vi "Anaysis Point Tool Histogram.vi"(0 "Pointer Listbox Detail":string[][](array[string]), 1 "Image":T1(plugin-control), 3 "Fixturing ROI":i32[](array[numeric]), 5 "error in":errorcluster) -> (14 "Pass/Fail":bool, 15 "Image":T1(plugin-control), 17 "Array":T2(array[cluster]), 19 "error out":errorcluster)   [LabVIEW 2020]
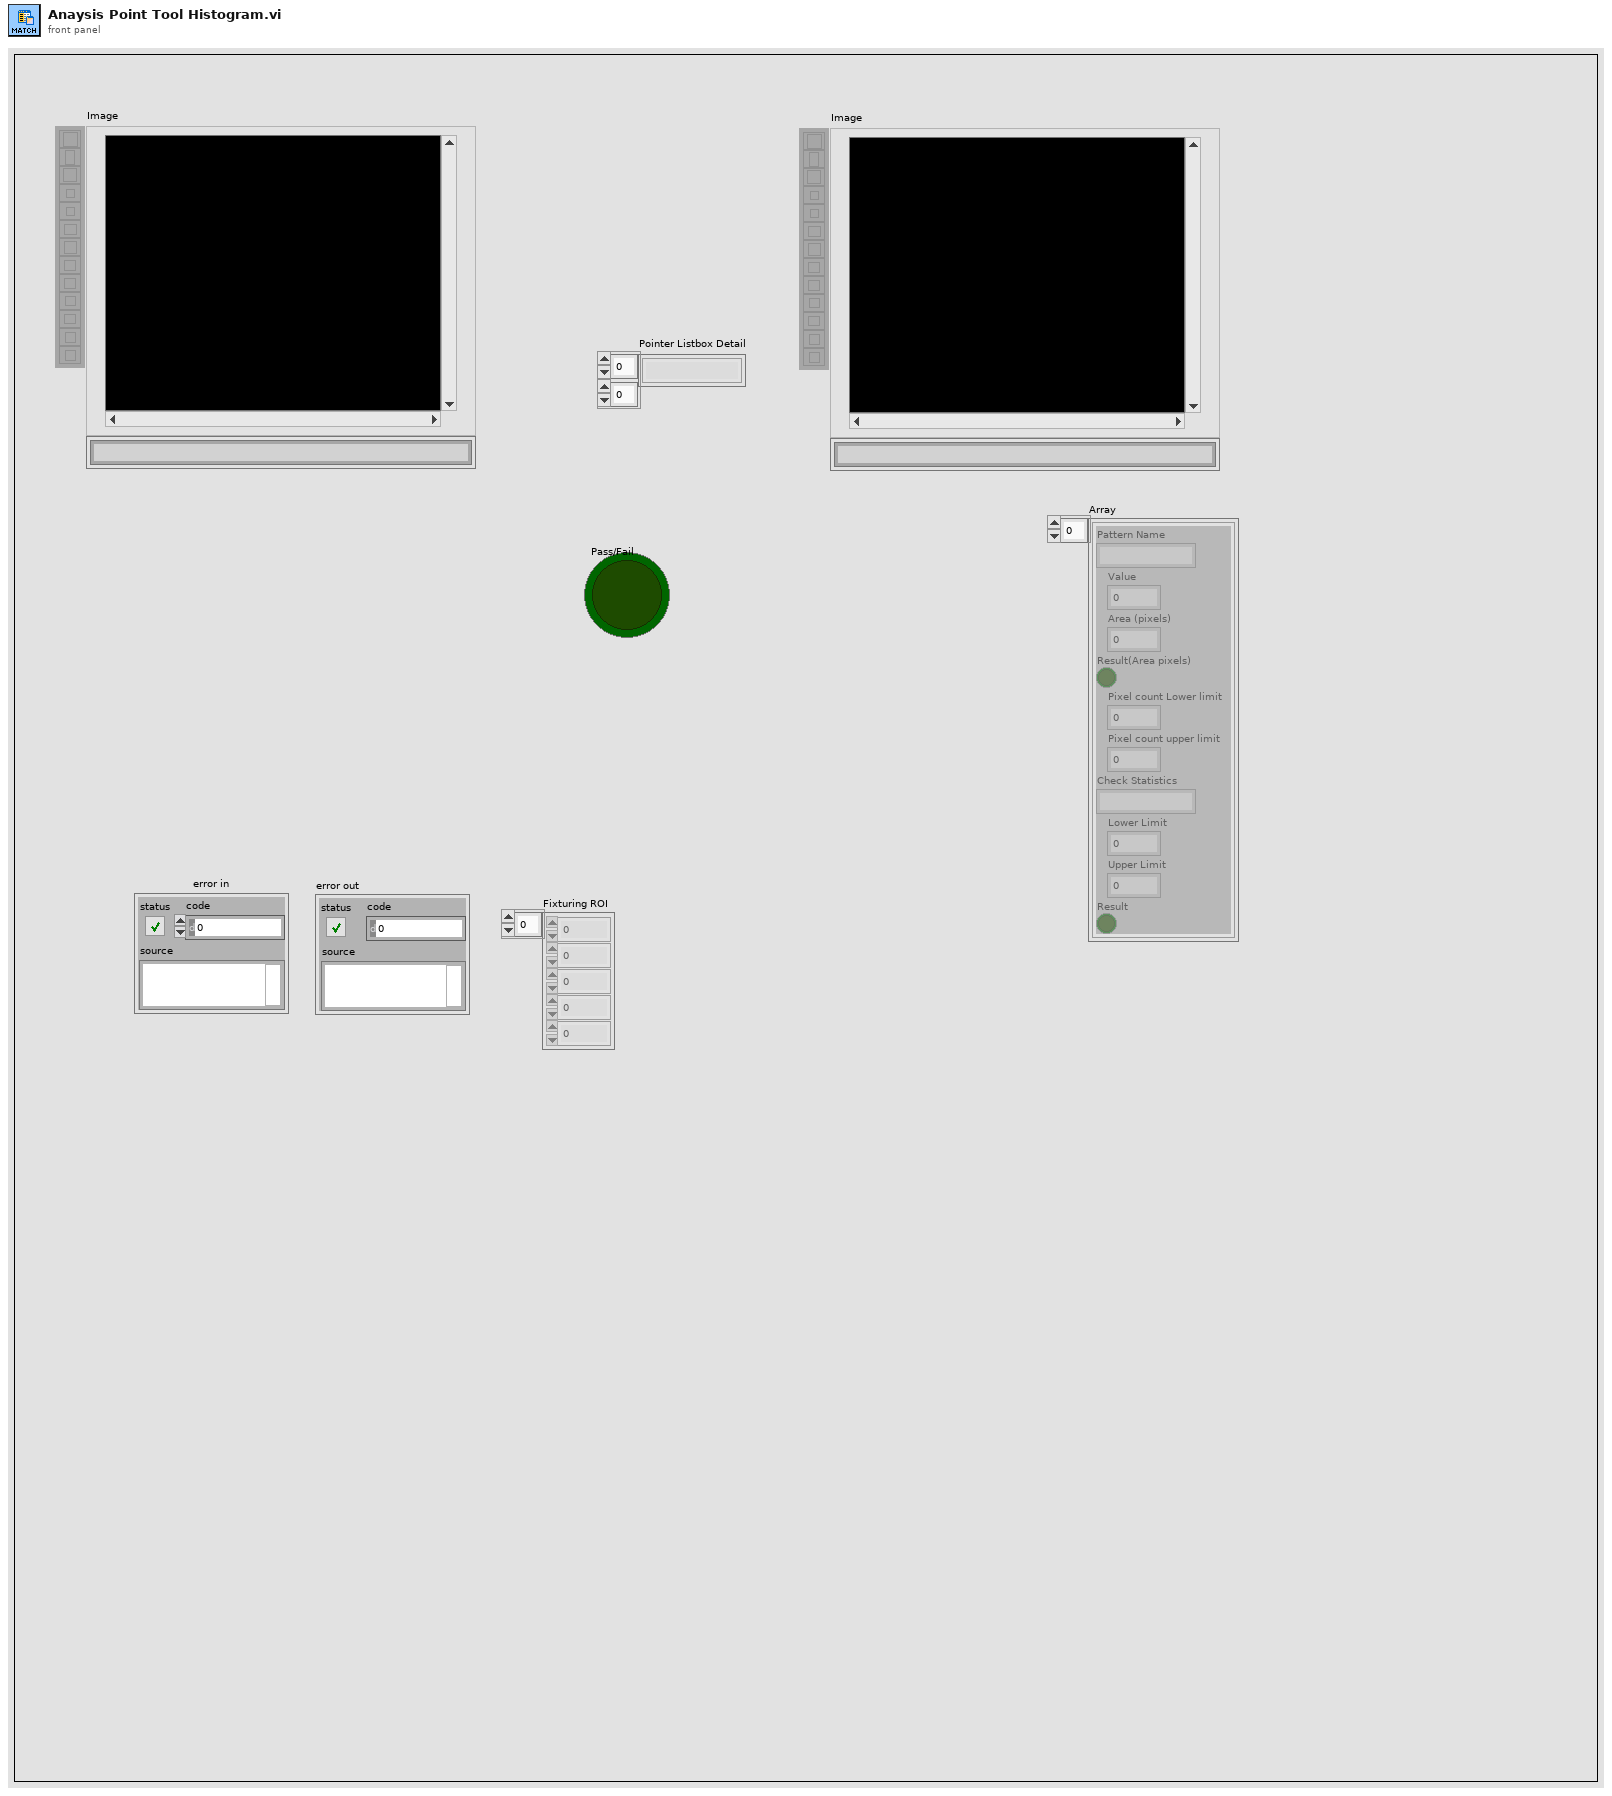
[diagram p1: front panel]
types:
  T1 = typedef "IMAQ Image.ctl" = refnum<image>
  T2 = cluster{"Pattern Name":string, "Value":ext, "Area (pixels)":i32, "Result(Area pixels)":bool, "Pixel count Lower limit":i32, "Pixel count upper limit":i32, "Check Statistics":string, "Lower Limit":i32, "Upper Limit":i32, "Result":bool}[]
  T3 = cluster{"Pixel count Lower limit":i32, "Pixel count upper limit":i32, "Check Statistics":string, "Lower Limit":i32, "Upper Limit":i32}
  T4 = cluster{"Global Rectangle":i32[], "Contours":cluster{"Contour Type":u32, "ROI Type":u32, "Points":i32[]}[]}
  T5 = cluster{"Global rect[0]":i32, "Global rect[1]":i32}
  T6 = cluster{i32[], cluster{"Contour Type":u32, "Contour Type":i32, i32[]}[]}
  T7 = cluster{"Minimal Value":sgl, "Maximal Value":sgl, "Mean Value":sgl, "Standard  Variation":sgl, "Area (pixels)":i32}
  T8 = typedef "ROI Descriptor" = cluster{"Global Rectangle":i32[], "Contours":cluster{"ID":enum32{"External", "Internal"}, "Type":u32, "Coordinates":i32[]}[]}
  T9 = cluster{"Rectangle out[0]":i32, "Rectangle out[1]":i32, "Rectangle out[2]":i32, "Rectangle out[3]":i32, "Rectangle out[4]":i32, "Rectangle out[5]":i32, "Rectangle out[6]":i32, "Rectangle out[7]":i32, "Rectangle out[8]":i32}
  T10 = cluster{"Rectangle out[0]":i32, "Rectangle out[1]":i32, "Rectangle out[2]":i32, "Rectangle out[3]":i32}
  T11 = cluster{"Pattern Name":string, "Value":ext, "Area (pixels)":i32, "Result(Area pixels)":bool, "Pixel count Lower limit":i32, "Pixel count upper limit":i32, "Check Statistics":string, "Lower Limit":i32, "Upper Limit":i32, "Result":bool}
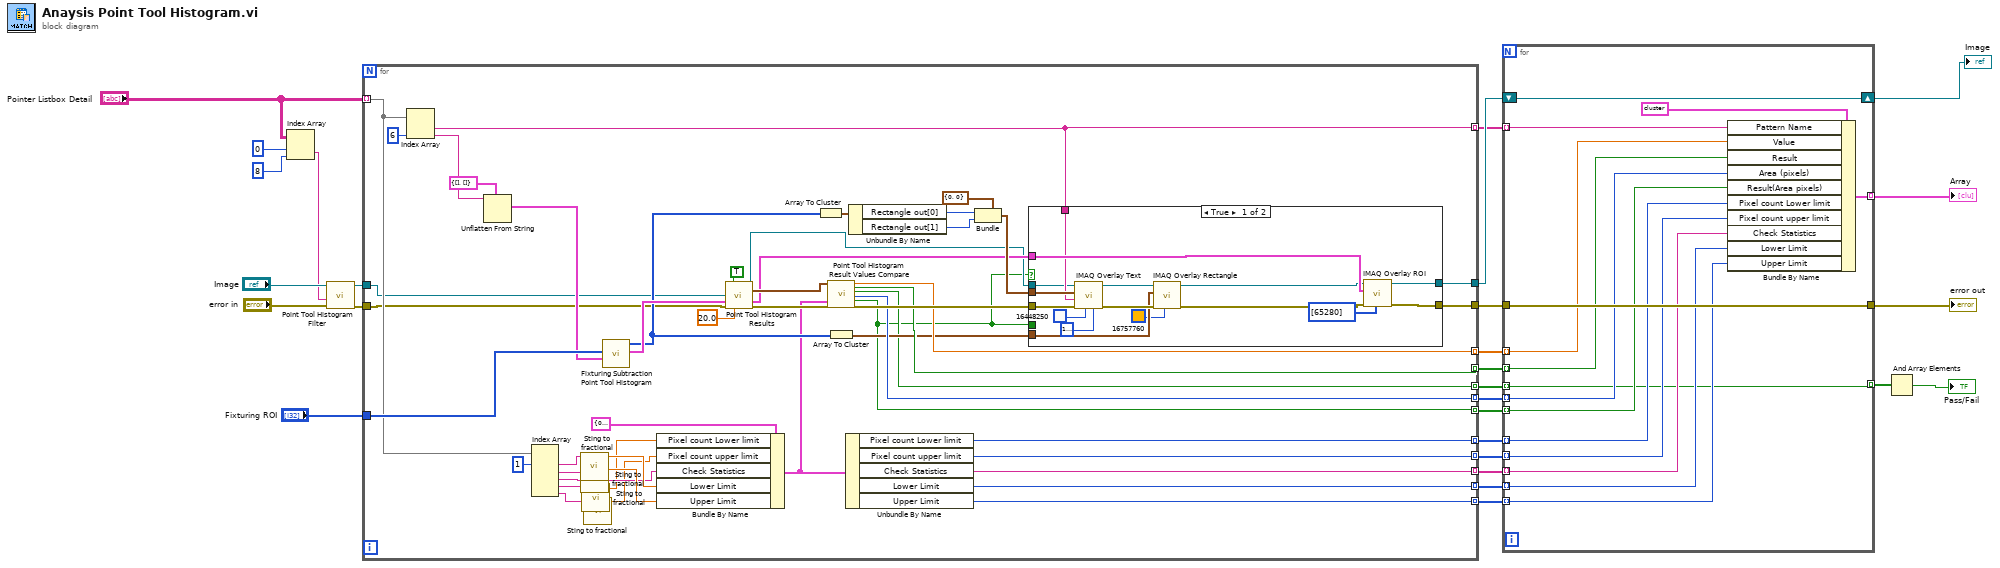
[diagram p0: block diagram]
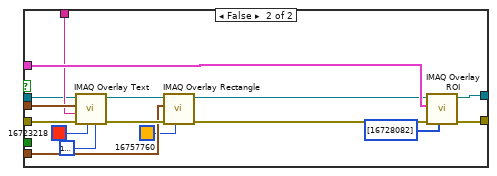
[diagram p2: hidden frame]
diagram:
  n1 = Index Array(array="Pointer Listbox Detail", index (row)=0 ("index"), index (col)=8 ("disabled index (col)")) -> (element=w3:string)
  n2 = call "Point Tool Histogram Filter.vi"("error in"="error in", "Combo Box"=w3, "Image in"="Image") -> ("error out"=w1:errorcluster, "Image out"=w4:T1)  [unwired: 7 in]
  n3 = for {
    tunnel: [w75] -> w27
    tunnel: w1 -> [w29]
    tunnel: [w62] -> w16 mode=indexing
    tunnel: [w50] -> w20 mode=indexing
    tunnel: [w61] -> w19 mode=indexing
    tunnel: [w28] -> w18 mode=indexing
    tunnel: [w60] -> w25 mode=indexing
    tunnel: [w59] -> w24 mode=indexing
    tunnel: [w58] -> w23 mode=indexing
    tunnel: [w57] -> w22 mode=indexing
    tunnel: [w56] -> w21 mode=indexing
    tunnel: [w55] -> w17 mode=indexing
    tunnel: "Fixturing ROI" -> [w53]
    tunnel: "Pointer Listbox Detail" -> [w44] mode=indexing
    tunnel: [w45] -> w9 mode=indexing
    tunnel: [w74] -> w15
    tunnel: w4 -> [w30]
    n4 = Index Array(array=w44, index #2=6 ("index")) -> (element #1=w45:string, element #2=w48:string)  [unwired: 1 in]
    n5 = Unflatten From String(type=T4 {"Global Rectangle"=[], "Contours"=[]} ("ROI"), binary string=w48) -> (value=w47:T4)  [unwired: 3 in, 2 out]
    n6 = Index Array(array=w44, index #1=1 ("index")) -> (element #1=w42:string, element #2=w40:string, element #3=w38:string, element #4=w36:string, element #5=w35:string)  [unwired: 4 in]
    n7 = call "Sting to fractional.vi"("String"=w42) -> ("Numeric"=w41:dbl)  [unwired: 10 in]
    n8 = call "Sting to fractional.vi"("String"=w40) -> ("Numeric"=w39:dbl)  [unwired: 10 in]
    n9 = call "Sting to fractional.vi"("String"=w36) -> ("Numeric"=w34:dbl)  [unwired: 10 in]
    n10 = call "Sting to fractional.vi"("String"=w35) -> ("Numeric"=w33:dbl)  [unwired: 10 in]
    n11 = call "Fixturing Subtraction Point Tool Histogram.vi"("ROI IN"=w47, "Fixturing ROI"=w53) -> ("ROI OUT"=w52:T6, "Rectangle out"=w51:i32[])  [unwired: 8 in]
    n12 = Bundle By Name(cluster=T3 {"Pixel count Lower limit"=0, "Pixel count upper limit"=0, "Check Statistics"="", "Lower Limit"=0, "Upper Limit"=0} ("input cluster"), "Pixel count Lower limit"=w34, "Pixel count upper limit"=w33, "Check Statistics"=w38, "Lower Limit"=w41, "Upper Limit"=w39) -> (w32:T3)
    n13 = call "Point Tool Histogram Results.vi"("Connectivity"=TRUE, "Main_Gray Out"=w30, "ROI"=w52, "error in"=w29, "Tolerance"=sgl 20.0) -> ("Refnum out"=w31:T1, "Statistics"=w69:T7, "ROI Descriptor"=w63:T8, "error out"=w71:errorcluster)  [unwired: 7 in]
    n14 = Array To Cluster(array=w51) -> (cluster=w68:T9)
    n15 = call "Point Tool Histogram Result Values Compare.vi"("Statistics"=w69, "Point Tool Histogram Limits"=w32, "error constant"=w71) -> ("Value"=w62:ext, "Result"=w55:bool, "Pass/Fail"=w50:bool, "Area (pixels)"=w61:i32, "Result(Area pixels)"=w28:bool, "error constant"=w70:errorcluster)  [unwired: 11 in]
    n16 = Array To Cluster(array=w51) -> (cluster=w54:T10)
    n17 = Unbundle By Name(w32) -> ("Pixel count Lower limit"=w60:i32, "Pixel count upper limit"=w59:i32, "Check Statistics"=w58:string, "Lower Limit"=w57:i32, "Upper Limit"=w56:i32)
    n18 = Unbundle By Name(w68) -> ("Rectangle out[0]"=w67:i32, "Rectangle out[1]"=w66:i32)
    n19 = Bundle(cluster=T5 {"Global rect[0]"=0, "Global rect[1]"=0}, "Global rect[0]"=w67, "Global rect[1]"=w66) -> (w64:T5)
    n20 = case shown="True" w28 {
      tunnel: [w91 w107] -> w75
      tunnel: [w90 w106] -> w74
      tunnel: w70 -> [w89 w105]
      tunnel: w64 -> [w88 w104]
      tunnel: w63 -> [w87 w103]
      tunnel: w28 -> [_ _]
      tunnel: w31 -> [w76 w92]
      tunnel: w54 -> [w82 w98]
      tunnel: w45 -> [w77 w93]
      frame True {
        n21 = call "IMAQ Overlay Text"("BG Color (Transparent)"=u32 16777228, "Text Color (black)"=u32 16448250, "error in (no error)"=w89, "String"=w77, "Origin"=w88, "Image"=w76) -> ("error out"=w84:errorcluster, "Image Out"=w81:T1)  [unwired: 4 in]
        n22 = call "IMAQ Overlay Rectangle"("Color"=u32 16757760, "error in (no error)"=w84, "Rectangle"=w82, "Image"=w81) -> ("error out"=w83:errorcluster, "Image Out"=w80:T1)  [unwired: 6 in]
        n23 = call "IMAQ Overlay ROI"("Colors (Green)"=u32[] [65280], "error in (no error)"=w83, "ROI Descriptor"=w87, "Image"=w80) -> ("error out"=w91:errorcluster, "Image Out"=w90:T1)  [unwired: 6 in]
      }
      frame False {
        n24 = call "IMAQ Overlay Text"("BG Color (Transparent)"=u32 16777228, "Text Color (black)"=u32 16723218, "error in (no error)"=w105, "String"=w93, "Origin"=w104, "Image"=w92) -> ("error out"=w100:errorcluster, "Image Out"=w97:T1)  [unwired: 4 in]
        n25 = call "IMAQ Overlay Rectangle"("Color"=u32 16757760, "error in (no error)"=w100, "Rectangle"=w98, "Image"=w97) -> ("error out"=w99:errorcluster, "Image Out"=w96:T1)  [unwired: 6 in]
        n26 = call "IMAQ Overlay ROI"("Colors (Green)"=u32[] [16728082], "error in (no error)"=w99, "ROI Descriptor"=w103, "Image"=w96) -> ("error out"=w107:errorcluster, "Image Out"=w106:T1)  [unwired: 6 in]
      }
    }
  }
  n27 = for {
    tunnel: [w121] -> w11 mode=indexing
    tunnel: w27 -> [w120]
    tunnel: [w120] -> w26
    tunnel: w25 -> [w116] mode=indexing
    tunnel: w24 -> [w115] mode=indexing
    tunnel: w23 -> [w114] mode=indexing
    tunnel: w22 -> [w113] mode=indexing
    tunnel: w21 -> [w112] mode=indexing
    tunnel: w20 -> [w109] mode=indexing
    tunnel: w19 -> [w117] mode=indexing
    tunnel: w18 -> [w111] mode=indexing
    tunnel: w17 -> [w118] mode=indexing
    tunnel: w16 -> [w119] mode=indexing
    tunnel: [w109] -> w13 mode=indexing
    tunnel: w9 -> [w108] mode=indexing
    shift-right: [w110] -> w14
    shift-left: w15 -> [w110]
    n28 = Bundle By Name(cluster=T11 {"Pattern Name"="", "Value"=0.0, "Area (pixels)"=0, "Result(Area pixels)"=FALSE, "Pixel count Lower limit"=0, "Pixel count upper limit"=0, "Check Statistics"="", "Lower Limit"=0, "Upper Limit"=0, "Result"=FALSE}, "Pattern Name"=w108, "Value"=w119, "Result"=w118, "Area (pixels)"=w117, "Result(Area pixels)"=w111, "Pixel count Lower limit"=w116, "Pixel count upper limit"=w115, "Check Statistics"=w114, "Lower Limit"=w113, "Upper Limit"=w112) -> (w121:T11)
  }
  "error out" <- w26
  "Image" <- w14
  "Array" <- w11
  n29 = And Array Elements(Boolean array=w13) -> (logical AND=→"Pass/Fail":bool)
